vi "Pitch Roll Calibration Loop.vi"() -> ()   [LabVIEW 2009]
uses:
  <vilib>/Platform/TimedLoop/XDataNode/XDataNode.xnode
  <vilib>/Platform/TimedLoop/XDataNode/loadlvalarms.vi
  <vilib>/Platform/TimedLoop/XDataNode/timing_clust.ctl
  <vilib>/Platform/TimedLoop/XDataNode/nitl_modes.ctl
  <vilib>/Platform/TimedLoop/XDataNode/wakeup.ctl
  Functional Global Variables/Actions for FG's.ctl
  <vilib>/Platform/TimedLoop/XDataNode/XDNodeRunTimeDep.lvlib
  <vilib>/Analysis/NI_AALBase.lvlib
panel:
  out "Roll":dbl(graph)
  out "Pitch":dbl(graph)
  out "Mean roll":dbl format="%0.2f"
  out "Average computed?":bool
  out "Mean pitch":dbl format="%0.2f"
  # "Mean pitch roll over 1 minute (2 samples per second)"
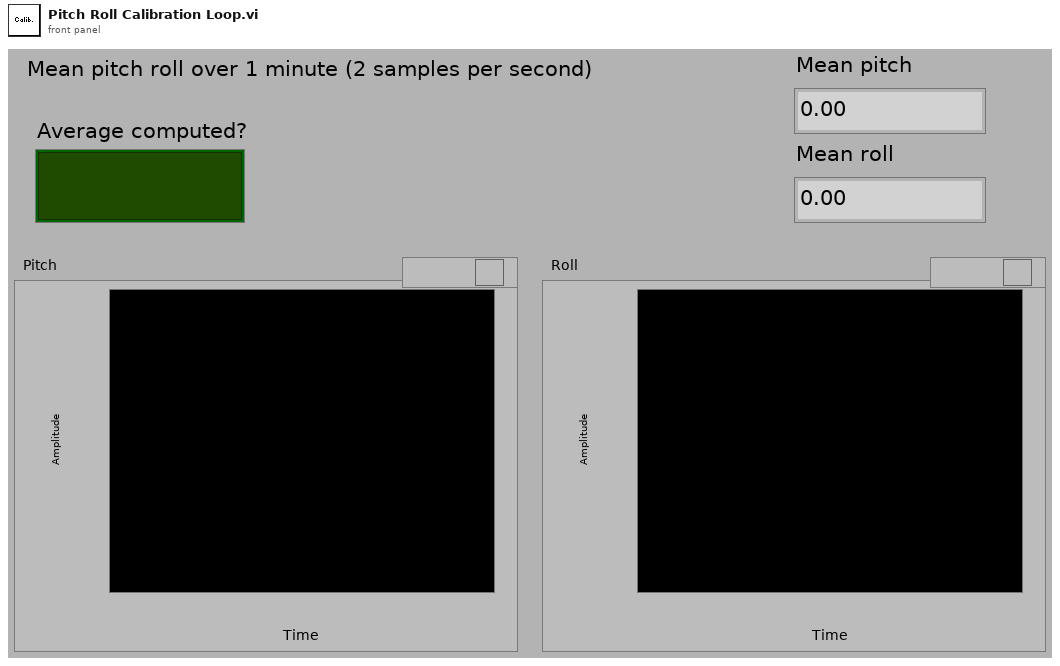
[diagram p1: front panel]
types:
  T1 = typedef "XDNodeRunTimeDep.lvlib/timing_clust.ctl" = cluster{"Expected End [f-1]":u64, "Actual End [f-1]":u64, "Finished Late? [f-1]":bool, "Expected End [i-1]":u64, "Actual End [i-1]":u64, "Finished Late? [i-1]":bool, "Expected Start [i]":u64, "Actual Start [i]":u64, "Expected Start [f]":u64, "Actual Start [f]":u64, "Source Name":string, "Structure Name":string, "Period":i64, "Deadline":i64, "Offset":i64, "Start":i64, "Priority":i32, "Timeout":i32, "Mode":T2, "Wakeup Reason":T3, "Error":errorcluster, "Source Type":string, "Secondary Source Type":string, "Global End Time":u64, "Global Start Time":u64, "Frame Duration":u64, "Iteration Duration":u64, "Assigned CPU":i32, "I/O Scan Engine Mode":u32}
  T2 = typedef "XDNodeRunTimeDep.lvlib/nitl_modes.ctl" = enum32{"No Change", "Process missed periods, maintain original phase", "Discard missed periods, maintain original phase", "Process missed periods, ignore original phase", "Discard missed periods, ignore original phase"}
  T3 = typedef "XDNodeRunTimeDep.lvlib/wakeup.ctl" = enum32{"Normal", "Aborted", "Asynchronous wakeup", "Timing source error", "Timed loop error", "Timeout"}
  T4 = typedef "Actions for FG's.ctl" = enum16{"Read", "Write"}
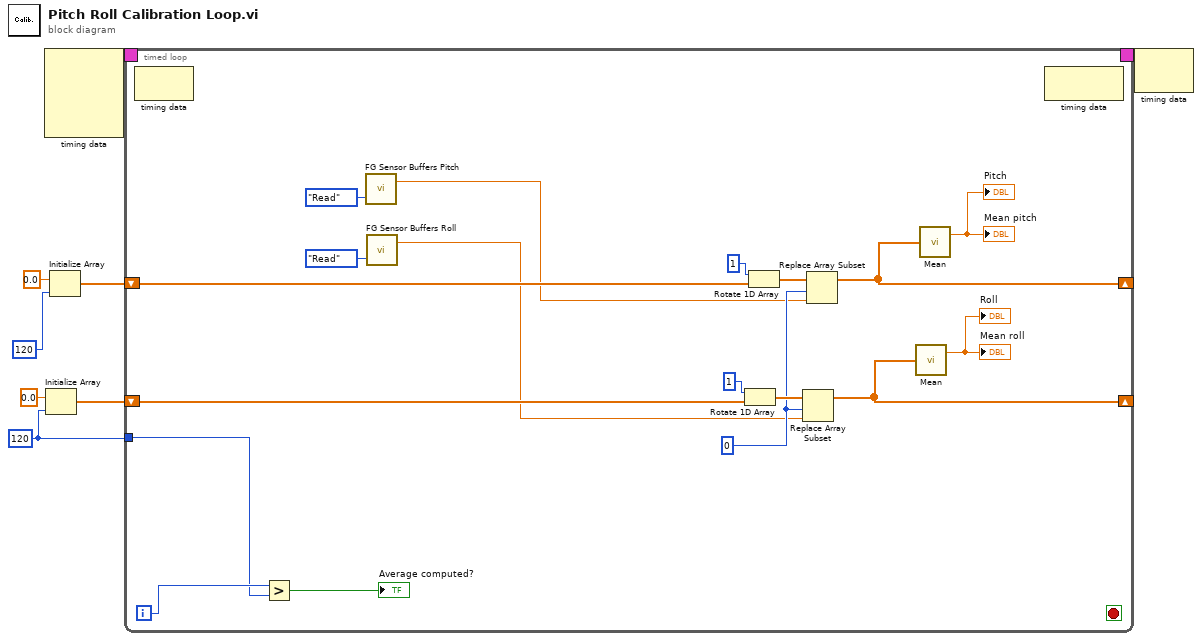
[diagram p0: block diagram]
diagram:
  w1 = 120 ("dimension size")
  n1 = node-c288() -> (w8:T1)  [unwired: 4 in]
  n2 = Initialize Array(0.0 ("element"), w1) -> (w3:dbl[])
  n3 = Initialize Array(0.0 ("element"), 120 ("dimension size")) -> (w5:dbl[])
  n4 = timed-loop {
    timing: w8 -> [_]
    timing-out: [_] -> w7
    shift-right: [w23] -> _
    shift-left: w5 -> [w24]
    tunnel: w1 -> [w18]
    shift-right: [w17] -> _
    shift-left: w3 -> [w16]
    i -> [w22]
    stop <- _ stop-if-true
    w13 = 0 ("index")
    n5 = node-c288() -> ()  [unwired: 1 in, 1 out]
    n6 = Greater?(x=w22, y=w18) -> (0:→"Average computed?":bool)
    n7 = call "FG Sensor Buffers Pitch.vi"("FG Action (Read)"=Actions_for_FG's."Read") -> ("Pitch Buffer out"=w11:dbl)  [unwired: 2 in]
    n8 = call "FG Sensor Buffers Roll.vi"("FG Action (Read)"=Actions_for_FG's."Read") -> ("Roll Buffer out"=w10:dbl)  [unwired: 2 in]
    n9 = Rotate 1D Array(1:w16, 2:1 ("n")) -> (0:w15:dbl[])
    n10 = Rotate 1D Array(1:w24, 2:1 ("n")) -> (0:w25:dbl[])
    n11 = Replace Array Subset(array=w15, new element=w10, index=w13) -> (w17:dbl[])
    n12 = Replace Array Subset(array=w25, new element=w11, index=w13) -> (w23:dbl[])
    n13 = call <vilib>:"Mean.vi"("X"=w17) -> ("mean"=→"Mean roll" →"Roll":dbl)  [unwired: 1 out]
    n14 = call <vilib>:"Mean.vi"("X"=w23) -> ("mean"=→"Mean pitch" →"Pitch":dbl)  [unwired: 1 out]
    n15 = node-c288() -> ()  [unwired: 1 in, 1 out]
  }
  n16 = node-c288(w7) -> ()  [unwired: 1 out]
